vi "pmu_Write Time Quality.vi"(8 "error in (no error)":errorcluster, 9 "unlocked time":u32, 10 "time quality flag":u8 format="%08b", 11 "system info in":refnum<class "PMU System Info.lvclass">) -> (0 "error out":errorcluster, 3 "system info out":refnum<class "PMU System Info.lvclass">)   [LabVIEW 2011, in "NI_EP_PMU.lvlib" / "PMU System Info.lvclass"]
uses:
  <vilib>/addons/Electrical Power/PMU/Common/Classes/PMU System Info/PMU System Info.lvclass
  <vilib>/addons/Electrical Power/PMU/Common/Classes/PMU System Info/PMU System Info.lvclass/PMU System Info.ctl
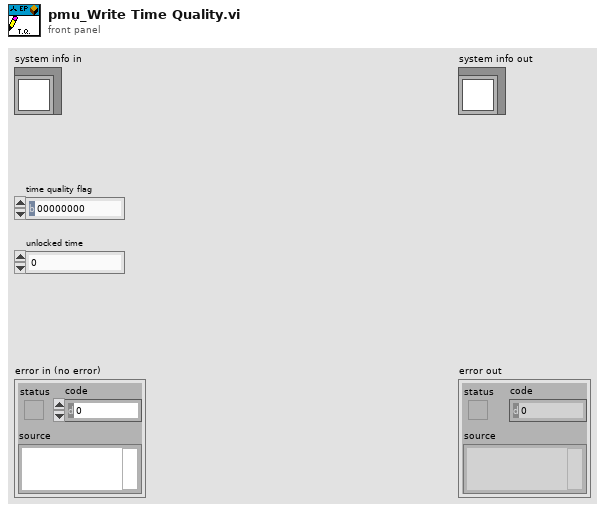
[diagram p1: front panel]
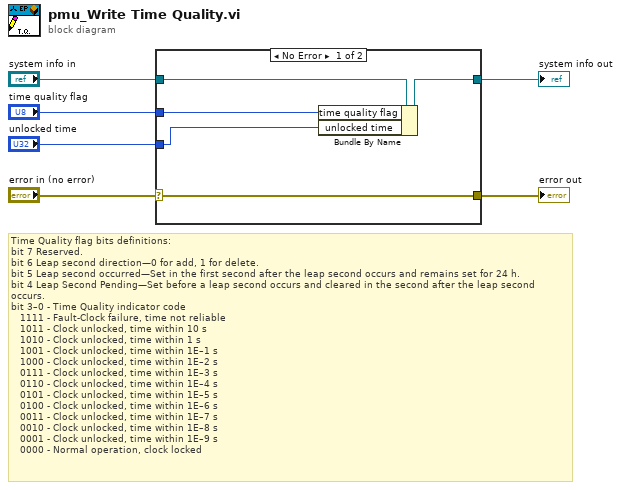
[diagram p0: block diagram]
diagram:
  # "Time Quality flag bits definitions:\nbit 7 Reserved.\nbit 6 Leap second direction—0 for add, 1 for delete.\nbit 5 Leap second occurred—Set in the first second after the leap second occurs and remains set for 24 h.\nbit 4 Leap Second Pending—Set before a leap second occurs and cleared in the second after the leap second occurs.\nbit 3–0 - Time Quality indicator code\n   1111 - Fault-Clock failure, time not reliable\n   1011 - Clock unlocked, time within 10 s\n   1010 - Clock unlocked, time within 1 s\n   1001 - Clock unlocked, time within 1E–1 s\n   1000 - Clock unlocked, time within 1E–2 s\n   0111 - Clock unlocked, time within 1E–3 s\n   0110 - Clock unlocked, time within 1E–4 s\n   0101 - Clock unlocked, time within 1E–5 s\n   0100 - Clock unlocked, time within 1E–6 s\n   0011 - Clock unlocked, time within 1E–7 s\n   0010 - Clock unlocked, time within 1E–8 s\n   0001 - Clock unlocked, time within 1E–9 s\n   0000 - Normal operation, clock locked"
  n1 = case shown="No Error" "error in (no error)" {
    selector: "error in (no error)" -> [w11 w12]
    tunnel: [w11 w12] -> w5
    tunnel: [w9 w13] -> w3
    tunnel: "system info in" -> [w10 w13]
    tunnel: "unlocked time" -> [w7 _]
    tunnel: "time quality flag" -> [w8 _]
    frame No Error {
      n2 = Bundle By Name(cluster=w10, "time quality flag"=w8, "unlocked time"=w7) -> (w9:refnum<class "PMU System Info.lvclass">)
    }
    frame Error {
    }
  }
  "error out" <- w5
  "system info out" <- w3
